vi "allocate_data_space.vi"(8 "error in (no error)":errorcluster, 11 "DAQmxWriteSignals in":refnum<class "SignalWriterDL090202DAQmx.lvclass">) -> (0 "error out":errorcluster, 3 "DAQmxWriteSignals out":refnum<class "SignalWriterDL090202DAQmx.lvclass">)   [LabVIEW 2010, in "SignalWriterDL090202DAQmx.lvclass"]
uses:
  SignalWriterDL090202DAQmx.lvclass
  common/enumerations/functional_global_action_enum.ctl
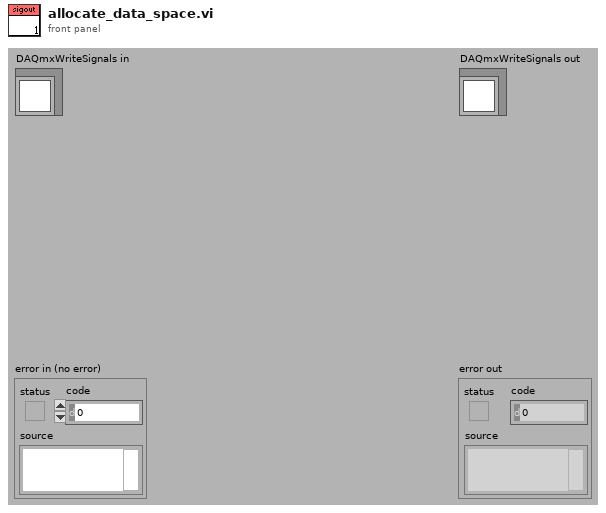
[diagram p1: front panel]
types:
  T1 = typedef "functional_global_action_enum.ctl" = enum16{"get", "set", "reset"}
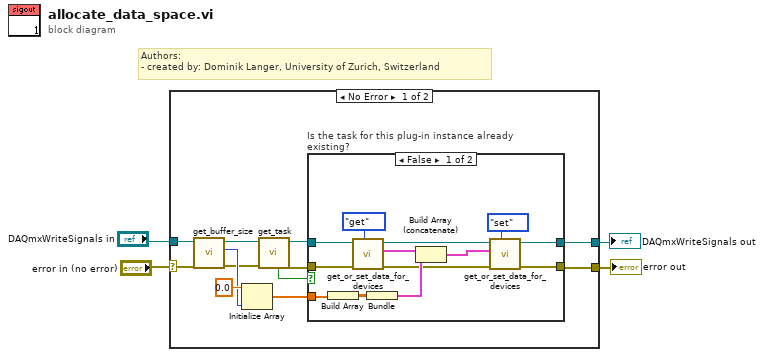
[diagram p0: block diagram]
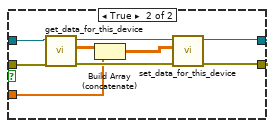
[diagram p2: hidden frame]
diagram:
  # "Authors: \n- created by: Dominik Langer, University of Zurich, Switzerland"
  n1 = case shown="No Error" "error in (no error)" {
    selector: "error in (no error)" -> [w10 w40]
    tunnel: [w15 w40] -> w1
    tunnel: [w16 w39] -> w4
    tunnel: "DAQmxWriteSignals in" -> [w9 w39]
    frame No Error {
      n2 = call-dynamic "get_buffer_size.vi"("error in (no error)"=w10, "GenericWriteSignals.lvclass in"=w9) -> ("error out"=w6:errorcluster, "buffer size (samples)"=w11:i32, "GenericWriteSignals.lvclass out"=w5:refnum<class "SignalWriterDL090202DAQmx.lvclass">)  [unwired: 7 out]
      n3 = Initialize Array(0.0 ("element"), w11) -> (w8:dbl[])
      n4 = call-dynamic "get_task.vi"("error in (no error)"=w6, "DAQmxWriteSignals in"=w5) -> ("error out"=w14:errorcluster, "DAQmxWriteSignals out"=w13:refnum<class "SignalWriterDL090202DAQmx.lvclass">, "found?"=w7:bool)  [unwired: 7 out]
      n5 = case "Is the task for this plug-in instance already existing?" shown="False" w7 {
        tunnel: w14 -> [w20 w32]
        tunnel: w13 -> [w21 w31]
        tunnel: [w27 w35] -> w16
        tunnel: [w26 w36] -> w15
        tunnel: w8 -> [w23 w30]
        frame False {
          n6 = Build Array(w23) -> (w29:dbl[][])
          n7 = call-dynamic "get_or_set_data_for_devices.vi"("action"=functional_global_action_enum."get", "error in (no error)"=w20, "DAQmxWriteSignals in"=w21) -> ("error out"=w19:errorcluster, "data for devices out"=w18:cluster{"data for channels":dbl[][]}[], "DAQmxWriteSignals out"=w17:refnum<class "SignalWriterDL090202DAQmx.lvclass">)  [unwired: 1 in, 5 out]
          n8 = Bundle(w29) -> (w28:cluster{dbl[][]})  [unwired: 1 in]
          n9 = Build Array (concatenate)(w18, w28) -> (w25:cluster{"data for channels":dbl[][]}[])
          n10 = call-dynamic "get_or_set_data_for_devices.vi"("action"=functional_global_action_enum."set", "error in (no error)"=w19, "data for devices in"=w25, "DAQmxWriteSignals in"=w17) -> ("error out"=w26:errorcluster, "DAQmxWriteSignals out"=w27:refnum<class "SignalWriterDL090202DAQmx.lvclass">)  [unwired: 6 out]
        }
        frame True {
          n11 = call-dynamic "get_data_for_this_device.vi"("error in (no error)"=w32, "DAQmxWriteSignals in"=w31) -> ("error out"=w37:errorcluster, "data"=w38:dbl[][], "DAQmxWriteSignals out"=w33:refnum<class "SignalWriterDL090202DAQmx.lvclass">)  [unwired: 7 out]
          n12 = Build Array (concatenate)(w38, w30) -> (w34:dbl[][])
          n13 = call-dynamic "set_data_for_this_device.vi"("error in (no error)"=w37, "data"=w34, "DAQmxWriteSignals in"=w33) -> ("error out"=w36:errorcluster, "DAQmxWriteSignals out"=w35:refnum<class "SignalWriterDL090202DAQmx.lvclass">)  [unwired: 7 out]
        }
      }
    }
    frame Error {
    }
  }
  "error out" <- w1
  "DAQmxWriteSignals out" <- w4
